vi "Update PID.vi"(8 "error in (no error)":errorcluster, 10 "ctl":cluster{"p":dbl, "i":dbl, "d":dbl}, 11 "Meerstetter TEC in":refnum<class "Meerstetter TEC.lvclass">) -> (0 "error out":errorcluster, 3 "Meerstetter TEC out":refnum<class "Meerstetter TEC.lvclass">)   [LabVIEW 2014, in "Meerstetter Lib.lvlib" / "Meerstetter TEC.lvclass"]
uses:
  Meerstetter TEC.lvclass
  Generic TEC/TEC.lvclass
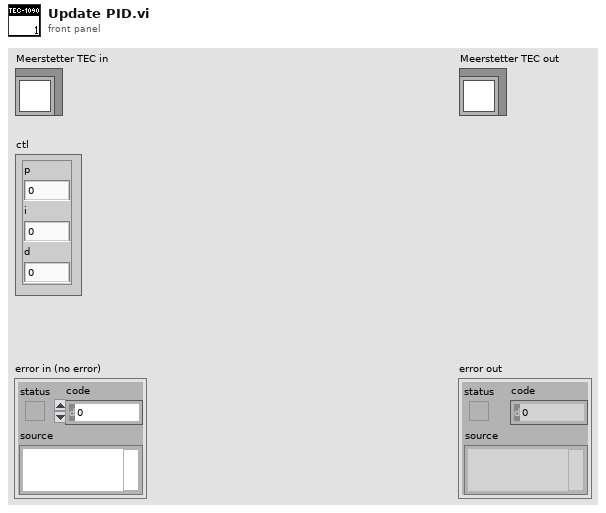
[diagram p1: front panel]
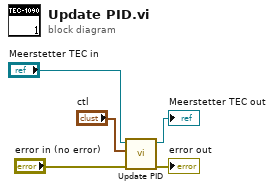
[diagram p0: block diagram]
diagram:
  n1 = call-parent "Update PID.vi"("error in (no error)"="error in (no error)", "ctl"="ctl", "TEC in"="Meerstetter TEC in") -> ("error out"=→"error out":errorcluster, "TEC out"=→"Meerstetter TEC out":refnum<class "Meerstetter TEC.lvclass">)  [unwired: 7 in]
